vi "Update FP Title.vi"(8 "error in (no error)":errorcluster, 10 "Cfg wChassis":T1, 11 "FP Controls in":refnum<class "FP Controls.lvclass">) -> (0 "error out":errorcluster, 3 "FP Controls out":refnum<class "FP Controls.lvclass">)   [LabVIEW 2018, in "Configuration Grandmaster.lvlib" / "FP Controls.lvclass"]
uses:
  FP Controls.lvclass
  Custom Ctrls/Master Cfg/ge_Cfg wChassis.ctl
  Class Chassis BOM/Chassis BOM.lvclass
  Class Chassis Cfg/ChassisCfg.lvclass
  Data Acquisition/Class Chassis Tasks/Chassis Tasks.lvclass
  FP Controls.lvclass/FP Controls.ctl
  Class Chassis BOM/Chassis BOM.lvclass/Chassis BOM.ctl
  Class Chassis BOM/Read Chassis Alias.vi
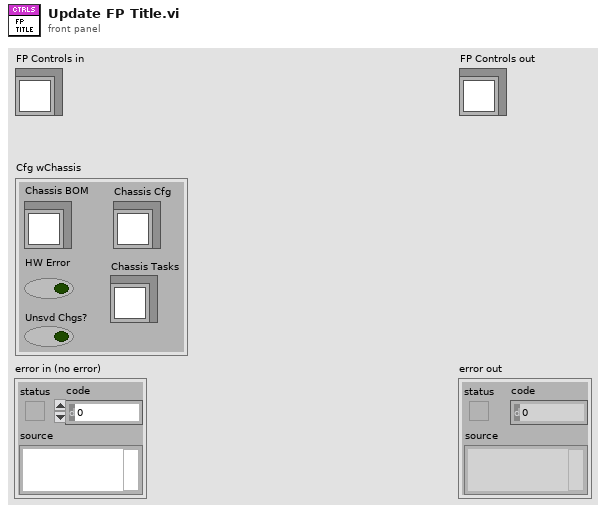
[diagram p1: front panel]
types:
  T1 = typedef "ge_Cfg wChassis.ctl" = cluster{"Chassis BOM":refnum<class "Chassis BOM.lvclass">, "Chassis Cfg":refnum<class "ChassisCfg.lvclass">, "Chassis Tasks":refnum<class "Chassis Tasks.lvclass">, "HW Error":bool, "Unsvd Chgs?":bool}
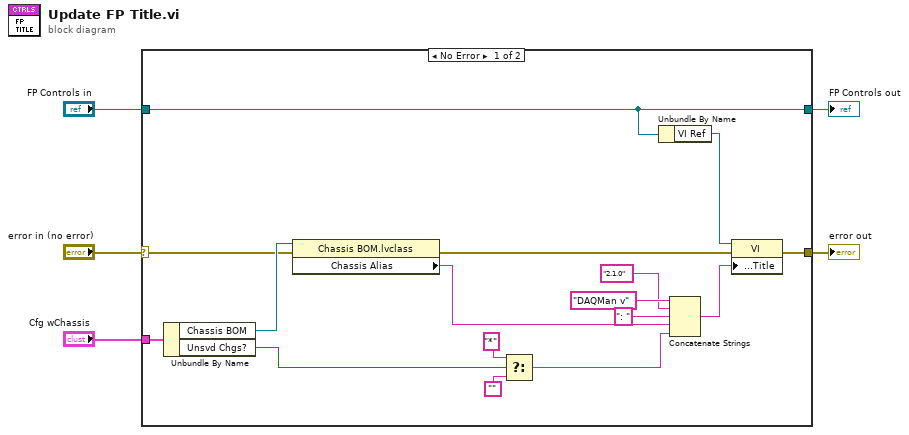
[diagram p0: block diagram]
diagram:
  n1 = case shown="No Error" "error in (no error)" {
    selector: "error in (no error)" -> [w8 w23]
    tunnel: [w18 w23] -> w4
    tunnel: [w17 w22] -> w2
    tunnel: "FP Controls in" -> [w17 w22]
    tunnel: "Cfg wChassis" -> [w12 _]
    frame No Error {
      n2 = Unbundle By Name(w12) -> ("Chassis BOM"=w15:refnum<class "Chassis BOM.lvclass">, "Unsvd Chgs?"=w9:bool)
      n3 = property class="Chassis BOM.lvclass"(reference=w15, error in=w8) -> (error out=w7:errorcluster, "Chassis Alias"=w11:string)  [unwired: 1 out]
      n4 = Select(t="*", s=w9, f="") -> (s? t:f=w10:string)
      n5 = Unbundle By Name(w17) -> ("VI Ref"=w16:refnum<vi>)
      n6 = Concatenate Strings("DAQMan v" ("string"), "2.1.0" ("string"), ": " ("string"), w11, w10) -> (w21:string)
      n7 = property class="VI"(reference=w16, error in=w7, "Front Panel.Title"=w21) -> (error out=w18:errorcluster)  [unwired: 1 out]
    }
    frame Error {
    }
  }
  "error out" <- w4
  "FP Controls out" <- w2
